vi "CreatingSubVI.vi"() -> ()   [LabVIEW 2024]
panel:
  in  "stop":bool
  out "Thermometer (C)":dbl
  in  "Temperature (F)":dbl
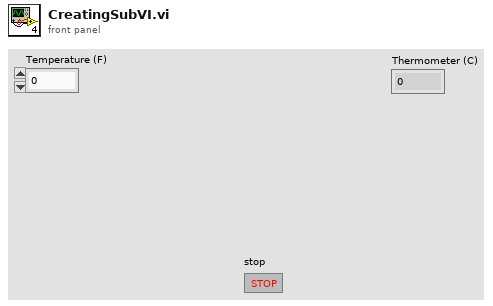
[diagram p1: front panel]
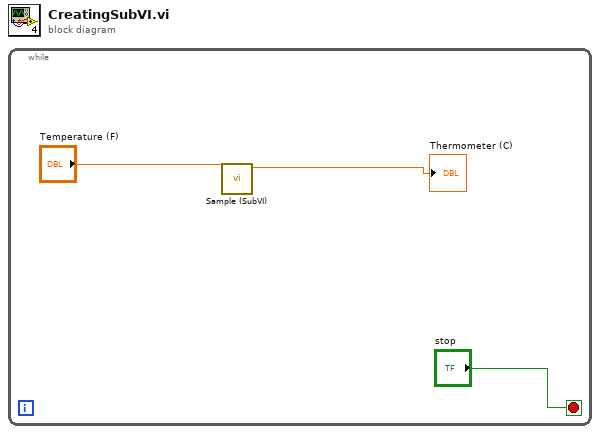
[diagram p0: block diagram]
diagram:
  n1 = while {
    stop <- "stop" stop-if-true
    n2 = call "Sample (SubVI).vi"("Temperature (F)"="Temperature (F)") -> ("Numeric"=→"Thermometer (C)":dbl)  [unwired: 10 in]
  }
